vi "CMI Sync V3 Set Channel 1 Division Factors.vi"(8 "error in":errorcluster, 9 "DDS multiplier (1)":i32=1, 10 "Divider (10)":i32=10, 11 "session in":T1={"VISA"="", "baud rate [bd/s]"=115200, "source"=enum."Auto", "hv range"=enum."1kV", "fsrc is fixed"=FALSE, "fsrc [Hz]"=10000000.0, "freq integ [s]"=1.0, "freq filter"=5, "trig level"=enum."TTL 5V", "chn1 mode"=enum."Source divider", "chn1 level"=enum."Positive 5V", "chn2 mode"=enum."Source divider", "chn2 level"=enum."Positive 5V", "chn2 div"=1, "chn3 mode"=enum."Chn 1 Active", "chn3 level"=enum."Positive 5V", "chn1 div entry"=enum."Calculate nearest divisor from measured fx", "chn1 dev limit [%]"=1.0, "chn1 check dev"=FALSE} {"chn2 div" min=1 max=100000000 step=1; "fsrc [Hz]" format="%_8p"}) -> (0 "error out":errorcluster, 3 "session out":T1={"VISA"="", "baud rate [bd/s]"=115200, "source"=enum."Auto", "hv range"=enum."1kV", "fsrc is fixed"=FALSE, "fsrc [Hz]"=10000000.0, "freq integ [s]"=1.0, "freq filter"=5, "trig level"=enum."TTL 5V", "chn1 mode"=enum."Source divider", "chn1 level"=enum."Positive 5V", "chn2 mode"=enum."Source divider", "chn2 level"=enum."Positive 5V", "chn2 div"=1, "chn3 mode"=enum."Chn 1 Active", "chn3 level"=enum."Positive 5V", "chn1 div entry"=enum."Calculate nearest divisor from measured fx", "chn1 dev limit [%]"=1.0, "chn1 check dev"=FALSE} {"chn2 div" min=1 max=100000000 step=1; "fsrc [Hz]" format="%_8p"})   [LabVIEW 2020, in "AWG.lvlib" / "CMI Sync Unit V3.lvlib"]
doc: "Sets output frequency of channel 1 (divisor, multiplier)."
uses:
  CMI Sync Unit V3.lvlib
  CMI Sync V3 session.ctl
  CMI Sync V3 Reference Clock Source.ctl
  CMI Sync V3 HV input Range.ctl
  CMI Sync V3 Trigger Input Level.ctl
  CMI Sync V3 Channel 1 Mode.ctl
  CMI Sync V3 Channel Output Levels.ctl
  CMI Sync V3 Channel 2 Mode.ctl
  CMI Sync V3 Channel 3 Mode.ctl
  CMI Sync V3 Channel 1 Divisor Entry Mode.ctl
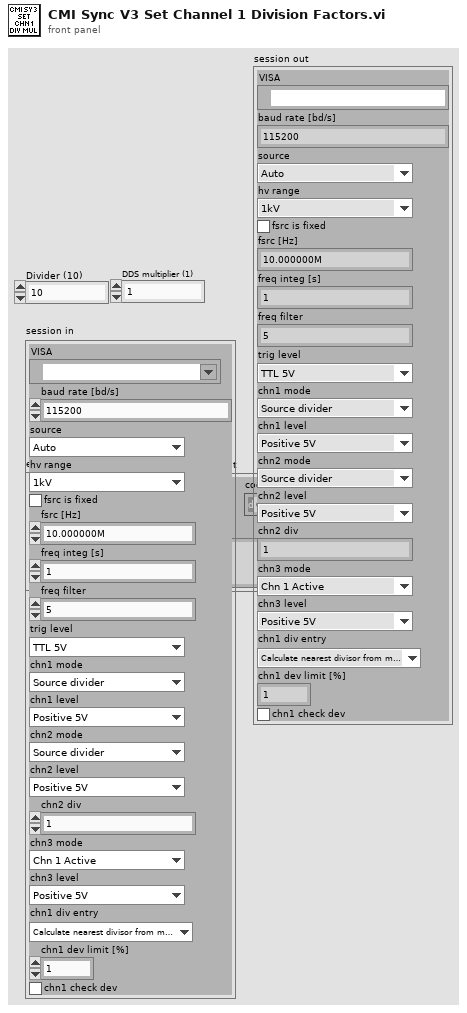
[diagram p1: front panel]
types:
  T1 = typedef "AWG.lvlib/CMI Sync Unit V3.lvlib/CMI Sync V3 session.ctl" = cluster{"VISA":refnum<visa-resource-name>, "baud rate [bd/s]":i32, "source":T2, "hv range":T3, "fsrc is fixed":bool, "fsrc [Hz]":dbl, "freq integ [s]":dbl, "freq filter":i32, "trig level":T4, "chn1 mode":T5, "chn1 level":T6, "chn2 mode":T7, "chn2 level":T6, "chn2 div":i32, "chn3 mode":T8, "chn3 level":T6, "chn1 div entry":T9, "chn1 dev limit [%]":dbl, "chn1 check dev":bool}
  T2 = typedef "AWG.lvlib/CMI Sync Unit V3.lvlib/CMI Sync V3 Reference Clock Source.ctl" = enum16{"Auto", "Internal", "Logic", "Sine", "HV"}
  T3 = typedef "AWG.lvlib/CMI Sync Unit V3.lvlib/CMI Sync V3 HV input Range.ctl" = enum16{"10V", "60V", "250V", "1kV"}
  T4 = typedef "AWG.lvlib/CMI Sync Unit V3.lvlib/CMI Sync V3 Trigger Input Level.ctl" = enum16{"LVCMOS 3V3", "TTL 5V"}
  T5 = typedef "AWG.lvlib/CMI Sync Unit V3.lvlib/CMI Sync V3 Channel 1 Mode.ctl" = enum16{"Source divider", "DDS absolute", "DDS ratio", "DDS ratio M/N"}
  T6 = typedef "AWG.lvlib/CMI Sync Unit V3.lvlib/CMI Sync V3 Channel Output Levels.ctl" = enum16{"Positive 3V3", "Negative 3V3", "Positive 5V", "Negative 5V"}
  T7 = typedef "AWG.lvlib/CMI Sync Unit V3.lvlib/CMI Sync V3 Channel 2 Mode.ctl" = enum16{"Source divider", "Chn 1 divide"}
  T8 = typedef "AWG.lvlib/CMI Sync Unit V3.lvlib/CMI Sync V3 Channel 3 Mode.ctl" = enum16{"Chn 1 Active", "Chn 2 Active", "Chn 1 Trigger", "Chn 2 Trigger", "Gate", "PPS", "10MHz"}
  T9 = typedef "AWG.lvlib/CMI Sync Unit V3.lvlib/CMI Sync V3 Channel 1 Divisor Entry Mode.ctl" = enum16{"Set divisor directly", "Calculate nearest divisor from measured fx"}
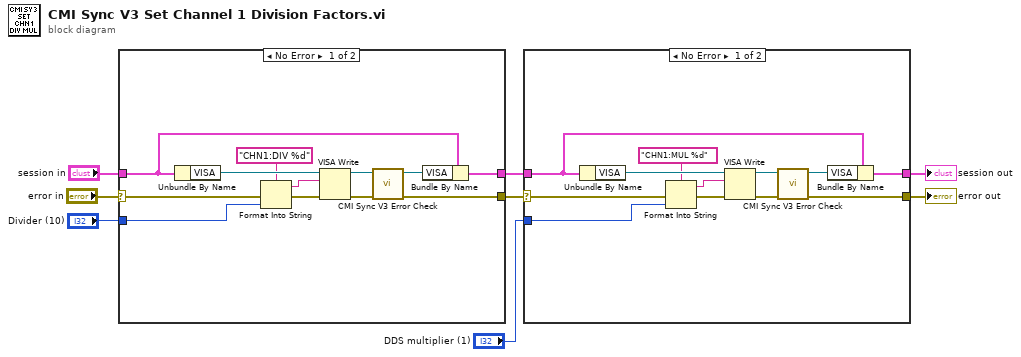
[diagram p0: block diagram]
diagram:
  n1 = case shown="No Error" "error in" {
    selector: "error in" -> [w13 w22]
    tunnel: "session in" -> [w20 w21]
    tunnel: [w19 w21] -> w4
    tunnel: [w14 w22] -> w5
    tunnel: "Divider (10)" -> [w9 _]
    frame No Error {
      n2 = Unbundle By Name(w20) -> ("VISA"=w18:refnum<visa-resource-name>)
      n3 = Format Into String(format string="CHN1:DIV %d", error in=w13, w9) -> (resulting string=w11:string, error out=w12:errorcluster)  [unwired: 1 in]
      n4 = VISA Write(VISA resource name=w18, write buffer=w11, error in (no error)=w12) -> (VISA resource name out=w16:refnum<visa-resource-name>, error out=w17:errorcluster)  [unwired: 1 out]
      n5 = call "CMI Sync V3 Error Check.vi"("error in"=w17, "VISA in"=w16) -> ("error out"=w14:errorcluster, "VISA out"=w15:refnum<visa-resource-name>)  [unwired: 7 in, 1 out]
      n6 = Bundle By Name(cluster=w20, "VISA"=w15) -> (w19:T1)
    }
    frame Error {
    }
  }
  n7 = case shown="No Error" w5 {
    selector: w5 -> [w27 w36]
    tunnel: w4 -> [w34 w35]
    tunnel: [w33 w35] -> w1
    tunnel: [w28 w36] -> w2
    tunnel: "DDS multiplier (1)" -> [w23 _]
    frame No Error {
      n8 = Unbundle By Name(w34) -> ("VISA"=w32:refnum<visa-resource-name>)
      n9 = Format Into String(format string="CHN1:MUL %d", error in=w27, w23) -> (resulting string=w25:string, error out=w26:errorcluster)  [unwired: 1 in]
      n10 = VISA Write(VISA resource name=w32, write buffer=w25, error in (no error)=w26) -> (VISA resource name out=w30:refnum<visa-resource-name>, error out=w31:errorcluster)  [unwired: 1 out]
      n11 = call "CMI Sync V3 Error Check.vi"("error in"=w31, "VISA in"=w30) -> ("error out"=w28:errorcluster, "VISA out"=w29:refnum<visa-resource-name>)  [unwired: 7 in, 1 out]
      n12 = Bundle By Name(cluster=w34, "VISA"=w29) -> (w33:T1)
    }
    frame Error {
    }
  }
  "error out" <- w2
  "session out" <- w1
